vi "Read Relight Point.vi"(8 "error in (no error)":errorcluster, 11 "BaseProducer in":refnum<class "BaseProducer.lvclass">) -> (0 "error out":errorcluster, 2 "Relight Point":dbl[](array[numeric]), 3 "BaseProducer out":refnum<class "BaseProducer.lvclass">)   [LabVIEW 2013, in "BaseProducer.lvclass"]
doc: "This method returns the relight state specified to the algoirthm."
uses:
  BaseProducer.lvclass
  BaseProducer.lvclass/BaseProducer.ctl
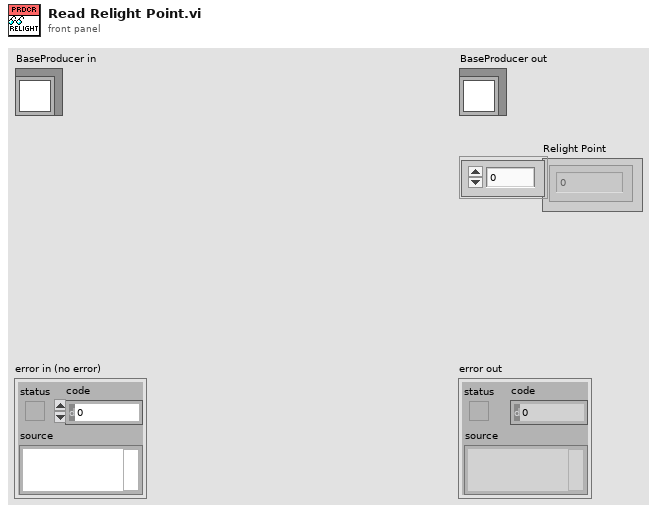
[diagram p1: front panel]
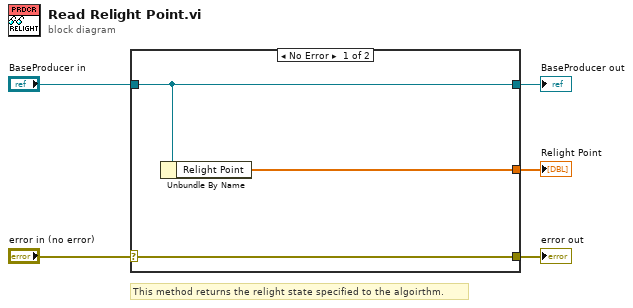
[diagram p0: block diagram]
diagram:
  # "This method returns the relight state specified to the algoirthm."
  n1 = case shown="No Error" "error in (no error)" {
    selector: "error in (no error)" -> [w8 w9]
    tunnel: [w8 w9] -> w4
    tunnel: [w7 w10] -> w2
    tunnel: "BaseProducer in" -> [w7 w10]
    tunnel: [w6 _] -> w1
    frame No Error {
      n2 = Unbundle By Name(w7) -> ("Relight Point"=w6:dbl[])
    }
    frame Error {
    }
  }
  "error out" <- w4
  "BaseProducer out" <- w2
  "Relight Point" <- w1
